vi "rs3_annotate_picture.vi"(4 "pixel center 2":cluster{"horizontal":i16, "vertical":i16}, 6 "Length":string="33.5", 8 "marker size":i16, 9 "pixel center1":cluster{"horizontal":i16, "vertical":i16}, 10 "Font size":i16, 11 "Input image":picture) -> (3 "new picture":picture)   [LabVIEW 2017, in "libRealSense3.lvlib"]
uses:
  libRealSense3.lvlib
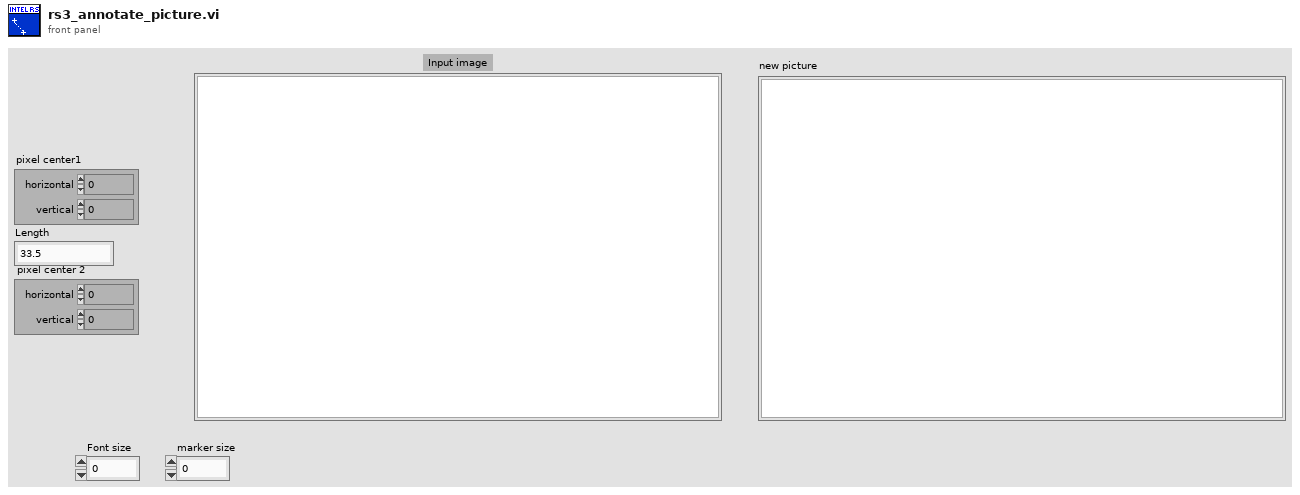
[diagram p1: front panel]
types:
  T1 = enum16{"User-specified Font", "Application Font", "System Font", "Dialog Font"}
  T2 = cluster{"Font Name:":string, "Size":i16, "Strikeout?":bool, "Italic?":bool, "Underline?":bool, "Outline?":bool, "Shadow?":bool, "Bold?":bool}
  T3 = cluster{"Width":u16, "Style":enum32{"Solid", "Dash", "Dot", "DashDot", "DashDotDot"}}
  T4 = cluster{"horizontal":enum16{"left", "center", "right"}, "vertical":enum16{"top", "center", "bottom"}}
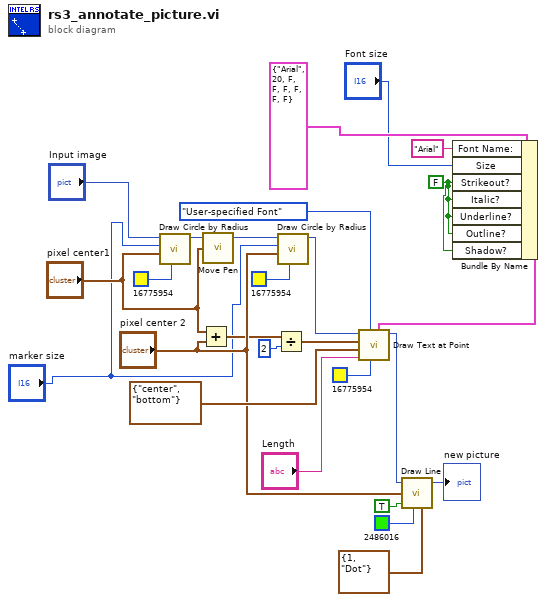
[diagram p0: block diagram]
diagram:
  w3 = FALSE ("Strikeout?")
  n1 = call <vilib>:"Draw Circle by Radius.vi"("color(black)"=u32 16775954, "pixel center"="pixel center1", "radius"="marker size", "picture"="Input image") -> ("new picture"=w18:picture)  [unwired: 7 in]
  n2 = Add(x="pixel center1", y="pixel center 2") -> (x+y=w10:cluster{"horizontal":i16, "vertical":i16})
  n3 = call <vilib>:"Move Pen.vi"("new position"="pixel center1", "picture"=w18) -> ("new picture"=w7:picture)  [unwired: 3 in]
  n4 = Divide(x=w10, y=i16 2 ("radius")) -> (x/y=w8:cluster{"horizontal":dbl, "vertical":dbl})
  n5 = call <vilib>:"Draw Circle by Radius.vi"("color(black)"=u32 16775954, "pixel center"="pixel center 2", "radius"="marker size", "picture"=w7) -> ("new picture"=w21:picture)  [unwired: 7 in]
  n6 = Bundle By Name(cluster=T2 {"Font Name:"="Arial", "Size"=20, "Strikeout?"=FALSE, "Italic?"=FALSE, "Underline?"=FALSE, "Outline?"=FALSE, "Shadow?"=FALSE, "Bold?"=FALSE} ("[user-specified font]"), "Font Name:"="Arial", "Size"="Font size", "Strikeout?"=w3, "Italic?"=w3, "Underline?"=w3, "Outline?"=w3, "Shadow?"=w3) -> (w2:T2)
  n7 = call <vilib>:"Draw Text at Point.vi"("[user-specified font]"=w2, "text color(black)"=u32 16775954, "desired font(Application)"=T1."User-specified Font", "text"="Length", "alignment(left, top)"=T4 {"horizontal"=enum."center", "vertical"=enum."bottom"}, "origin"=w8, "picture"=w21) -> ("new picture"=w22:picture)  [unwired: 3 in, 1 out]
  n8 = call <vilib>:"Draw Line.vi"("picture"=w22, "end point"="pixel center 2", "absolute coordinates?(T)"=TRUE, "color(black)"=u32 2486016, "pen"=T3 {"Width"=1, "Style"=enum."Dot"}) -> ("new picture"=→"new picture":picture)  [unwired: 4 in]
